vi "sound.vi"   [LabVIEW 2014]
types:
  T1 = typedef "Sound Output Task ID.ctl" = u32
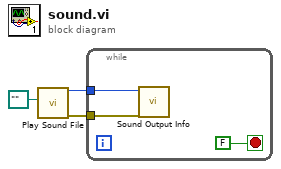
[diagram p0: block diagram]
diagram:
  n1 = call <vilib>:"Play Sound File.vi"("path"=path "") -> ("error out"=w2:errorcluster, "task ID"=w3:T1)  [unwired: 9 in]
  n2 = while {
    tunnel: w3 -> [w6]
    tunnel: w2 -> [w5]
    stop <- FALSE stop-if-true
    n3 = call <vilib>:"Sound Output Info.vi"("error in (no error)"=w5, "task ID"=w6) -> ()  [unwired: 6 in, 4 out]
  }
